vi "BRig_Host_dataRunState_dataPlot_reward3.vi"() -> (2 "output_idx_dataPlot_reward3":i32)   [LabVIEW 2014]
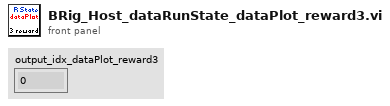
[diagram p1: front panel]
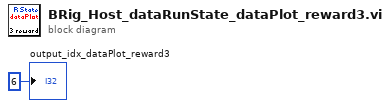
[diagram p0: block diagram]
diagram:
  "output_idx_dataPlot_reward3" <- 6 ("output_idx_dataTS")
